vi "Video-to-Array-Convert-first5images.vi"() -> ()   [LabVIEW 2012]
uses:
  <vilib>/Utility/file.llb/Write To Spreadsheet File (I64).vi
panel:
  out "Image Pixels (U8)":u8[][](array[numeric])
  in  "stop":bool
  out "Frames":T1(plugin-control)
  out "framesPerSecond":u32
  out "Image Type":T2 items=["Grayscale (U8)", "Grayscale (I16)", "Grayscale (SGL)", "Complex (CSG)", "RGB (U32)", "HSL (U32)", "RGB (U64)"]
  out "Number of Frames":u32
  in  "Path":path=path "C:/Users/admin/Desktop/lohit/pat3.avi"
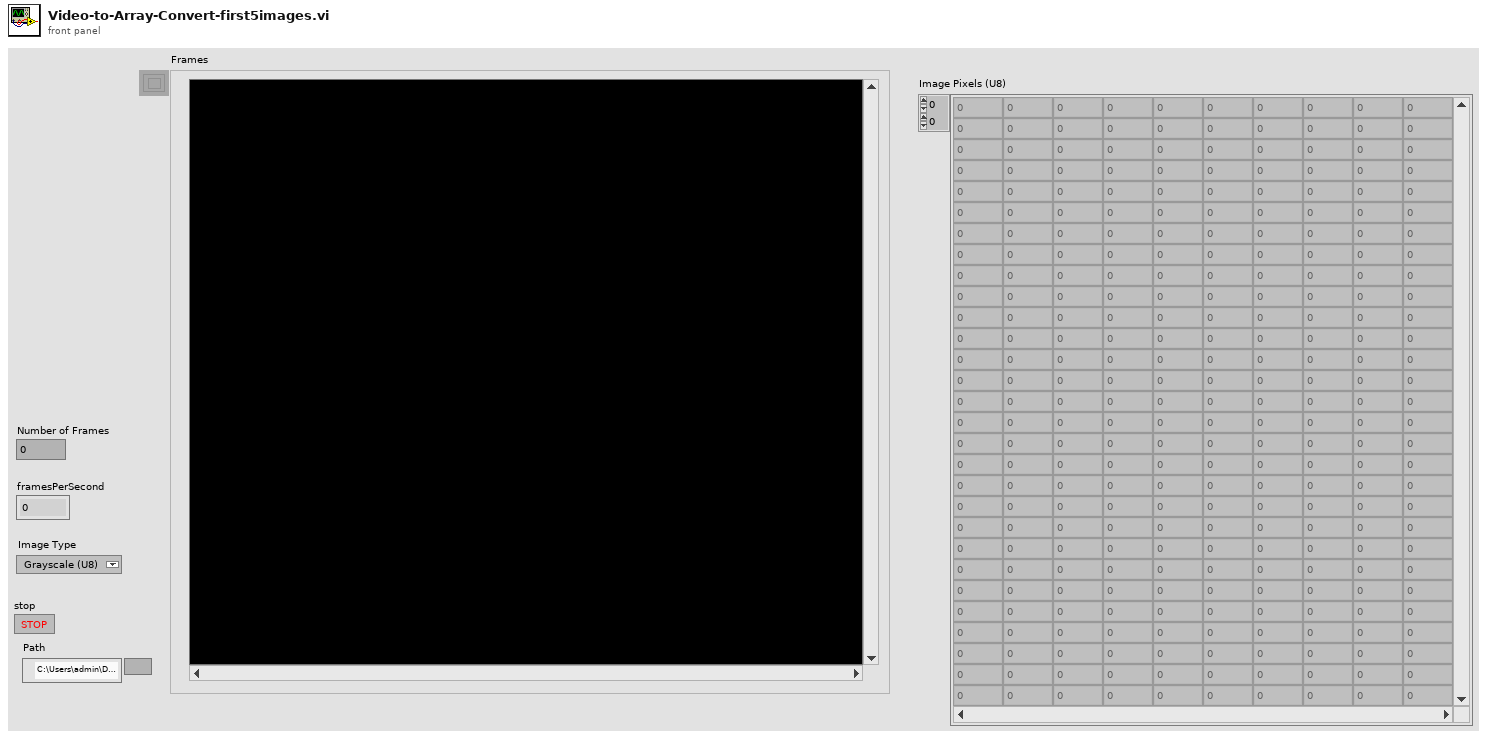
[diagram p1: front panel]
types:
  T1 = typedef "IMAQ Image.ctl" = refnum<image>
  T2 = typedef "Image Type" = u32
  T3 = typedef "AviRefnum.ctl" = refnum<k1>
  T4 = cluster{"width":u32, "height":u32, "framesPerSecond":u32, "compressionFilter":string, "hasData":bool}
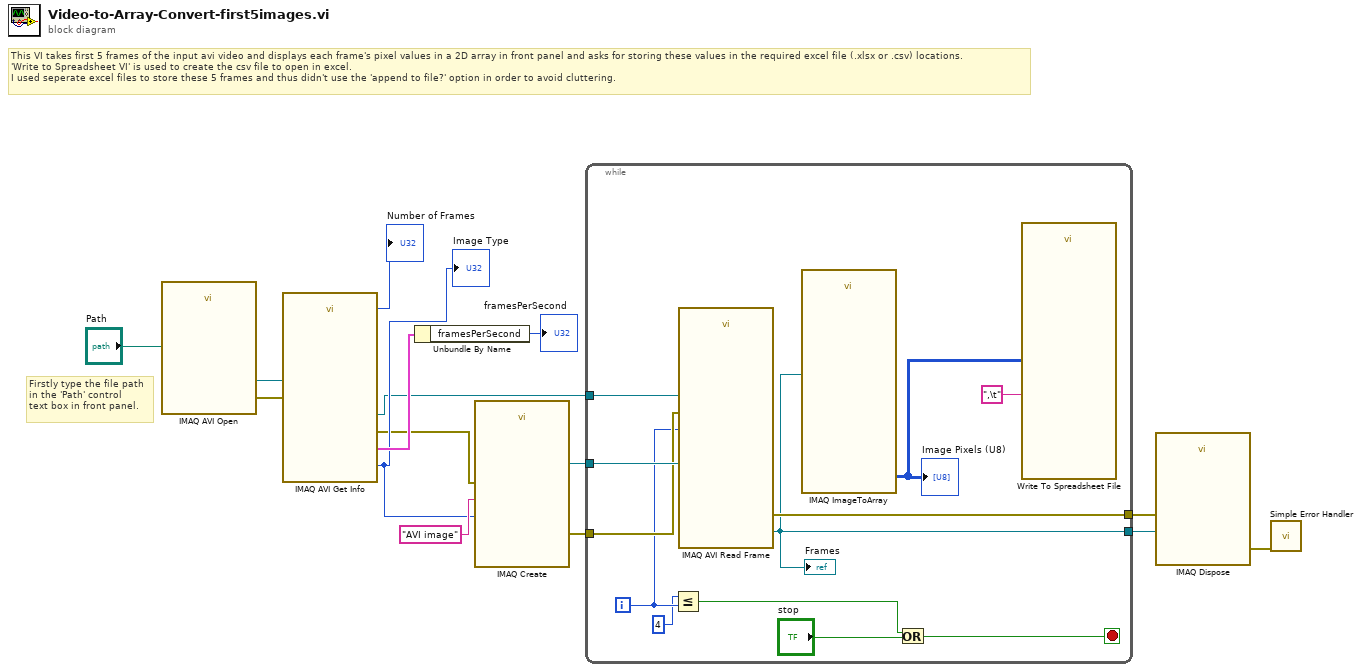
[diagram p0: block diagram]
diagram:
  # "Firstly type the file path\nin the 'Path' control \ntext box in front panel."
  # "This VI takes first 5 frames of the input avi video and displays each frame's pixel values in a 2D array in front panel and asks for storing these values in the required excel file (.xlsx or .csv) locations.\n'Write to Spreadsheet VI' is used to create the csv file to open in excel.\nI used seperate excel files to store these 5 frames and thus didn't use the 'append to file?' option in order to avoid cluttering."
  n1 = call "IMAQ AVI Open"("AVI Path"="Path") -> ("error out"=w8:errorcluster, "Avi Refnum"=w14:T3)  [unwired: 9 in]
  n2 = call "IMAQ AVI Get Info"("error in (no error)"=w8, "Avi Refnum"=w14) -> ("error out"=w7:errorcluster, "Image Type"=w10:T2, "Number of Frames"=→"Number of Frames":u32, "Avi Refnum (duplicate)"=w4:T3, "Frame Data"=w12:T4)  [unwired: 5 in]
  "Image Type" <- w10
  n3 = Unbundle By Name(w12) -> ("framesPerSecond"=→"framesPerSecond":u32)
  n4 = call "IMAQ Create"("Image Name"="AVI image", "Image Type"=w10, "error in (no error)"=w7) -> ("New Image"=w5:T1, "error out"=w3:errorcluster)  [unwired: 2 in]
  n5 = while {
    tunnel: w5 -> [w27]
    tunnel: w4 -> [w26]
    tunnel: w3 -> [w25]
    tunnel: [w18] -> w2
    tunnel: [w19] -> w1
    i -> [w24]
    stop <- w21 stop-if-true
    n6 = Less Or Equal?(x=u32 4 ("y"), y=w24) -> (x <= y?=w20:bool)
    n7 = call "IMAQ AVI Read Frame"("error in (no error)"=w25, "Frame Number"=w24, "Image"=w27, "Avi Refnum"=w26) -> ("error out"=w19:errorcluster, "Image Out"=w18:T1)  [unwired: 4 in, 2 out]
    "Frames" <- w18
    n8 = call "IMAQ ImageToArray"("Image"=w18) -> ("Image Pixels (U8)"=w17:u8[][])  [unwired: 3 in, 4 out]
    "Image Pixels (U8)" <- w17
    n9 = Or(x=w20, y="stop") -> (x .or. y?=w21:bool)
    n10 = call-poly <vilib>:"Write To Spreadsheet File.vi"("delimiter (\\t)"=",\t" ("delimiter (\\t)"), "2D data"=w17) -> ()  [unwired: 6 in, 1 out]
  }
  n11 = call "IMAQ Dispose"("Image"=w2, "error in (no error)"=w1) -> ("error out"=w6:errorcluster)  [unwired: 4 in]
  n12 = call <vilib>:"Simple Error Handler.vi"("error in (no error)"=w6) -> ()  [unwired: 4 in, 5 out]
